vi "ADXRS453_Init.vi"(10 "SPI Bus":T3=enum."SPI On-Board, CS2") -> (0 "Error Out":errorcluster, 2 "Gyro Detected?":bool, 3 "ADXRS453 Ref Out":T1)   [LabVIEW 2014]
doc: "ADXRS453 SPI Gyro\n\nThis example shows how to use the ADXRS453 Gyro sensor connected to SPI.\n\nThis example expects a USB cable connected from your development PC to the Type B USB Jack (next to the power input) on the roboRIO."
uses:
  <vilib>/Rock Robotics/SystemInterfaces/spilib/spi_bus.ctl
  <vilib>/Rock Robotics/WPI/SPI/WPI_SPIDevRef.ctl
  <vilib>/Rock Robotics/SystemInterfaces/Typedef/FPGA_TypedefDigitalModule.ctl
  <vilib>/Rock Robotics/WPI/Gyro/ADXRS453/WPI_Gyro_ADXRS453_Registers.ctl
  <vilib>/Rock Robotics/WPI/SPI/WPI_SPIMode.ctl
panel:
  # "This shows wiring for the Analog Devices ADXRS453 Gyro."
  # "Gryo"
  # "ADXRS453\nCS (blue)--------\nMISO (yellow)--\nMOSI (green)---\nCLK (orange)---\nPDD (red)-------\nGND (black)----"
  # "roboRIO\nSPI    CS1\nSPI    MISO\nSPI    MOSI\nSPI    SCLK\nSPI    5V\nSPI"
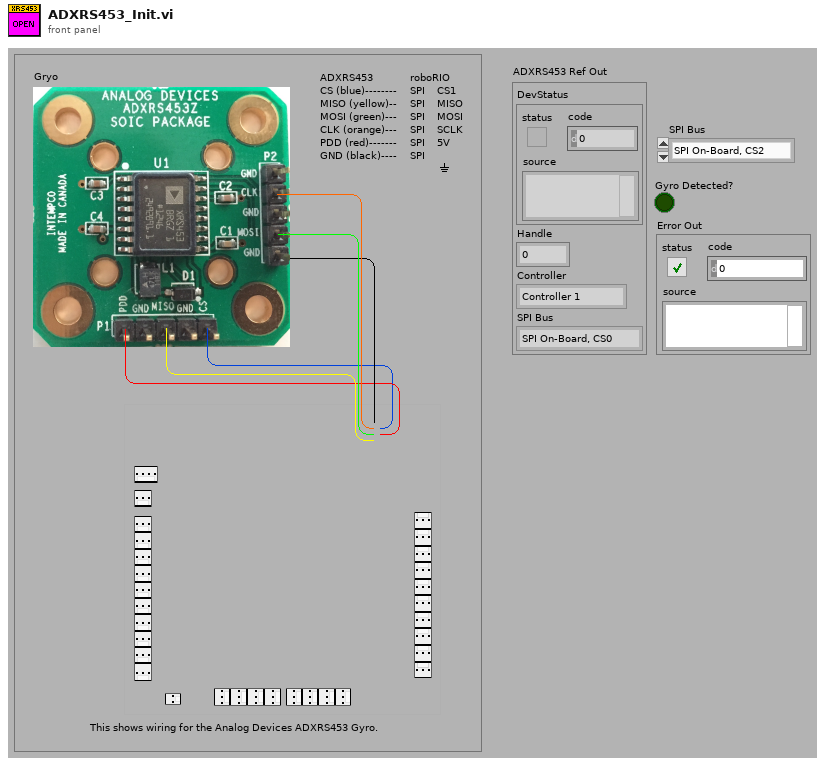
[diagram p1: front panel]
types:
  T1 = typedef "WPI_SPIDevRef.ctl" = cluster{"DevStatus":errorcluster, "Handle":i32, "Controller":T2, "SPI Bus":T3}
  T2 = typedef "FPGA_TypedefDigitalModule.ctl" = enum16{"Controller 1"}
  T3 = typedef "spi_bus.ctl" = enum16{"SPI On-Board, CS0", "SPI On-Board, CS1", "SPI On-Board, CS2", "SPI On-Board, CS3", "SPI MXP", "Invalid"}
  T4 = typedef "WPI_SPIMode.ctl" = enum16{"Mode 0 (Clk Idle Low,Sample on Leading)", "Mode 1 (Clk Idle Low,Sample on Trailing)", "Mode 2 (Clk Idle High,Sample on Leading)", "Mode 3 (Clk Idle High,Sample on Trailing)"}
  T5 = typedef "WPI_Gyro_ADXRS453_Registers.ctl" = u16
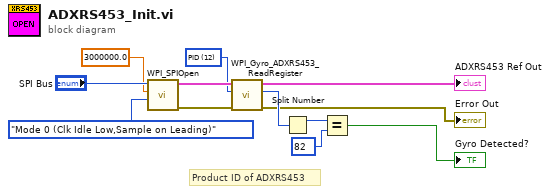
[diagram p0: block diagram]
diagram:
  w10 = T5 12 items=["Rate"=0, "Tem"=2, "LoCST"=4, "HiCST"=6, "Quad"=8, "Fault"=10, "PID"=12, "SN High"=14, "SN Low"=16]
  # "Product ID of ADXRS453"
  n1 = call <vilib>:"WPI_SPIOpen.vi"("Mode (3)"=WPI_SPIMode."Mode 0 (Clk Idle Low,Sample on Leading)", "Clock Rate (Hz)"=3000000.0, "SPI Bus"="SPI Bus") -> ("error out"=w8:errorcluster, "SPIDevRef"=w11:T1)  [unwired: 3 in, 4 out]
  n2 = call <vilib>:"WPI_Gyro_ADXRS453_ReadRegister.vi"("error in (no error)"=w8, "ADXRS453 Register"=w10, "SPIDevRef in"=w11) -> ("error out"=→"Error Out":errorcluster, "Register Value"=w6:u16, "SPIDevRef out"=→"ADXRS453 Ref Out":T1)  [unwired: 6 in]
  n3 = Split Number(x=w6) -> (hi(x)=w5:u8)  [unwired: 1 out]
  n4 = Equal?(x=w5, y=u8 82) -> (x = y?=→"Gyro Detected?":bool)
